vi "ConfigureDlg.vi"(8 "error in (no error)":errorcluster, 11 "ArbitraryFunction in":refnum<class "ArbitraryFunction.lvclass">) -> (0 "error out":errorcluster, 2 "Changed":bool, 3 "ArbitraryFunction out":refnum<class "ArbitraryFunction.lvclass">)   [LabVIEW 2018, in "Functions.lvlib" / "ArbitraryFunction.lvclass"]
uses:
  ArbitraryFunction.lvclass
  FunctionBaseClass/FunctionBase.lvclass
panel:
  # "No configurable Parameters for this Function"
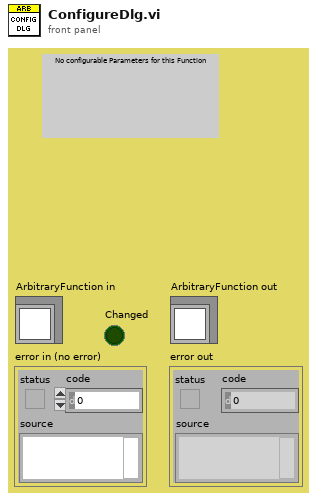
[diagram p1: front panel]
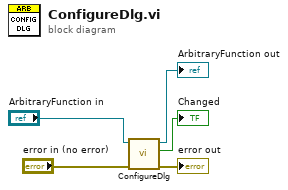
[diagram p0: block diagram]
diagram:
  n1 = call-parent "ConfigureDlg.vi"("error in (no error)"="error in (no error)", "FunctionBase in"="ArbitraryFunction in") -> ("error out"=→"error out":errorcluster, "Changed"=→"Changed":bool, "FunctionBase out"=→"ArbitraryFunction out":refnum<class "ArbitraryFunction.lvclass">)  [unwired: 7 in]
